vi "get Active Device.vi"(11 "Memory Map in":refnum<class "Memory Map.lvclass">) -> (3 "Active Device":T1)   [LabVIEW 2021, in "Memory Map.lvclass"]
uses:
  Memory Map.lvclass
  Active Device.ctl
  Memory Map.lvclass/Memory Map.ctl
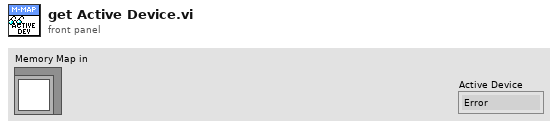
[diagram p1: front panel]
types:
  T1 = typedef "Memory Map.lvclass/Active Device.ctl" = enum16{"Error", "None", "RAM", "EEPROM", "VIA"}
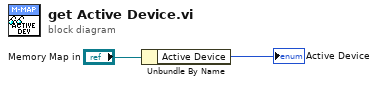
[diagram p0: block diagram]
diagram:
  n1 = Unbundle By Name("Memory Map in") -> ("Active Device"=→"Active Device":T1)
